vi "VisionUI.vi"() -> ()   [LabVIEW 2019]
uses:
  Ctrl/Snap.ctl
  Ctrl/Grab.ctl
  Ctrl/VisionProcessName.ctl
  Ctrl/UpDate.ctl
  Ctrl/Photo.ctl
  iVision/Analysis/Controls/V_Analysis_Type.ctl
  Ctrl/Calibration2.ctl
  <vilib>/vision/Image Controls.llb/IMAQ Image.ctl
  <vilib>/Utility/miscctls.llb/LVPointTypeDef.ctl
  <vilib>/Utility/miscctls.llb/LVPositionTypeDef.ctl
  iVision/Controls/Parameter.ctl
  LLB/Message/Ctrl/MsgDataInput.ctl
  LLB/Message/Ctrl/MsgPageSelect.ctl
  LLB/Message/Ctrl/LogType.ctl
  ccd1199d-ef2c-458d-9c2f-56e76543a288.vi
  ee1b8d73-df58-408e-9e82-1fda4488e2bc.vi
  7c6cd57d-ca9a-43cf-ba35-76cd5e228dea.vi
  c26e9516-a3f7-4664-a029-1caed30bc8c5.vi
  1dbde9c2-a06a-4c94-bdcc-a34a29a424c7.vi
  0675717f-6bf9-442b-96fb-61433deac2ff.vi
  bb48f479-1741-454e-9e2e-b2767c3551b8.vi
  488a8706-5b30-4d61-98bf-6c761bf059b6.vi
  687379a0-31af-4f7e-a561-925614dc81ac.vi
  a72d5238-090f-4a71-aba8-2c37060f7c47.vi
  74253ac0-82c8-4d34-a7ac-78c8919cb84d.vi
  340a900b-8271-4ea1-897c-4e5630e46489.vi
  8373cba2-dfce-4ae2-bf55-a53a2c69f5d3.vi
  <vilib>/JDP Science/JSONtext/Variant to JSON Text.vi
  LLB/Commonly VI/Main Glb.vi
  iVision/Global/VisionGlb.vi
  Class/Main Process Class/MPC_VirbVision/Panel RefGlb.vi
  <vilib>/JDP Science/JSONtext/JSON text to Variant.vi
  LLB/Commonly VI.lvlib
  <vilib>/vision/NI_Vision_Development_Module.lvlib
  LLB/Message/MsgShowAndLog.lvlib
panel:
  in  "Btn_Result Remove":bool
  in  "Btn_ResultAdd":bool
  in  "OutPutList":i32(listbox) caption="輸出列表"
  in  "Btn_Calibration":T1
  out "Calibration Axis Info":T2={"Origin Pixel"={"X"=0.0, "Y"=0.0}, "Angle Relative to Horizontal (deg)"=0.0, "X Axis Pixel"={"X"=0.0, "Y"=0.0}, "Axis Reference"=1} {"X Axis Pixel"."Y" format="%.2f"; "X Axis Pixel"."X" format="%.2f"; "Axis Reference" items=["Direct", "Indirect"]; "Angle Relative to Horizontal (deg)" format="%.2f"; "Origin Pixel"."Y" format="%.2f"; "Origin Pixel"."X" format="%.2f"}
  out "Grid Descriptor":T3={"X Step"=1.0, "Y Step"=1.0, "Unit"=enum."Undefined"} {"Y Step" format="%.2f"; "X Step" format="%.2f"}
  out "Calibration Done":bool
  in  "Btn_RemoveAlgorithm":bool
  in  "Btn_Add Algorithm":bool
  in  "AlgParameter":string
  in  "Algorithm List":i32(listbox)
  in  "SubUI":bool=TRUE
  out "PreProcess2":T5=enum."G_Threshold"
  in  "Btn_Load":bool
  out "Root Path":path
  in  "DataTable":T6(array[cluster])
  in  "Enum_Algorithm":enum16{"CG_Histogram", "C_Color Matching"}(ring)
  in  "Tab Control":enum32{"Page 1", "Page 2"}(tab)
  in  "Btn_ROITryrun":bool
  in  "Tab Control 3":enum32{"SetProcess", "ROI結果"}(tab)
  in  "Tab Control 2":enum32{"Process", "Algorithm", "Result"}(tab)
  in  "Btn_Test":bool
  out "Image 2":T7(plugin-control)
  in  "Enum_PreProcess":T5
  in  "Btn_RemovePreProcess":bool
  in  "Btn_Add PreProcess":bool
  in  "Process List":i32(listbox)
  in  "Algorithm":T8=enum."C_Color Pattern Matching"
  out "Image 3":T7(plugin-control)
  in  "Btn_TestAlg":bool
  in  "Btn_SetAlg":bool
  in  "Result":i32(listbox) caption="結果清單"
  in  "Btn_RenewROIData":T9
  in  "ROIOutPutList All":i32(listbox) caption="全部結果"
  in  "Photo":T10
  in  "Btn_DelProject":bool
  in  "Btn_AddProject":bool
  in  "Btn_EditROI":bool
  in  "Btn_DelROI":bool
  in  "Btn_AddROI":bool
  in  "btn_Grab":T11
  in  "Btn_Snap":T12
  in  "List ROI":i32(listbox)
  in  "Btn_Save":bool
  in  "ProjectSet":u16(ring) caption="設定資料"
  out "Image":T7(plugin-control)
  in  "相機":u16(ring) items=["cam0"]
  # "P_:Pixel\nR_RealWord"
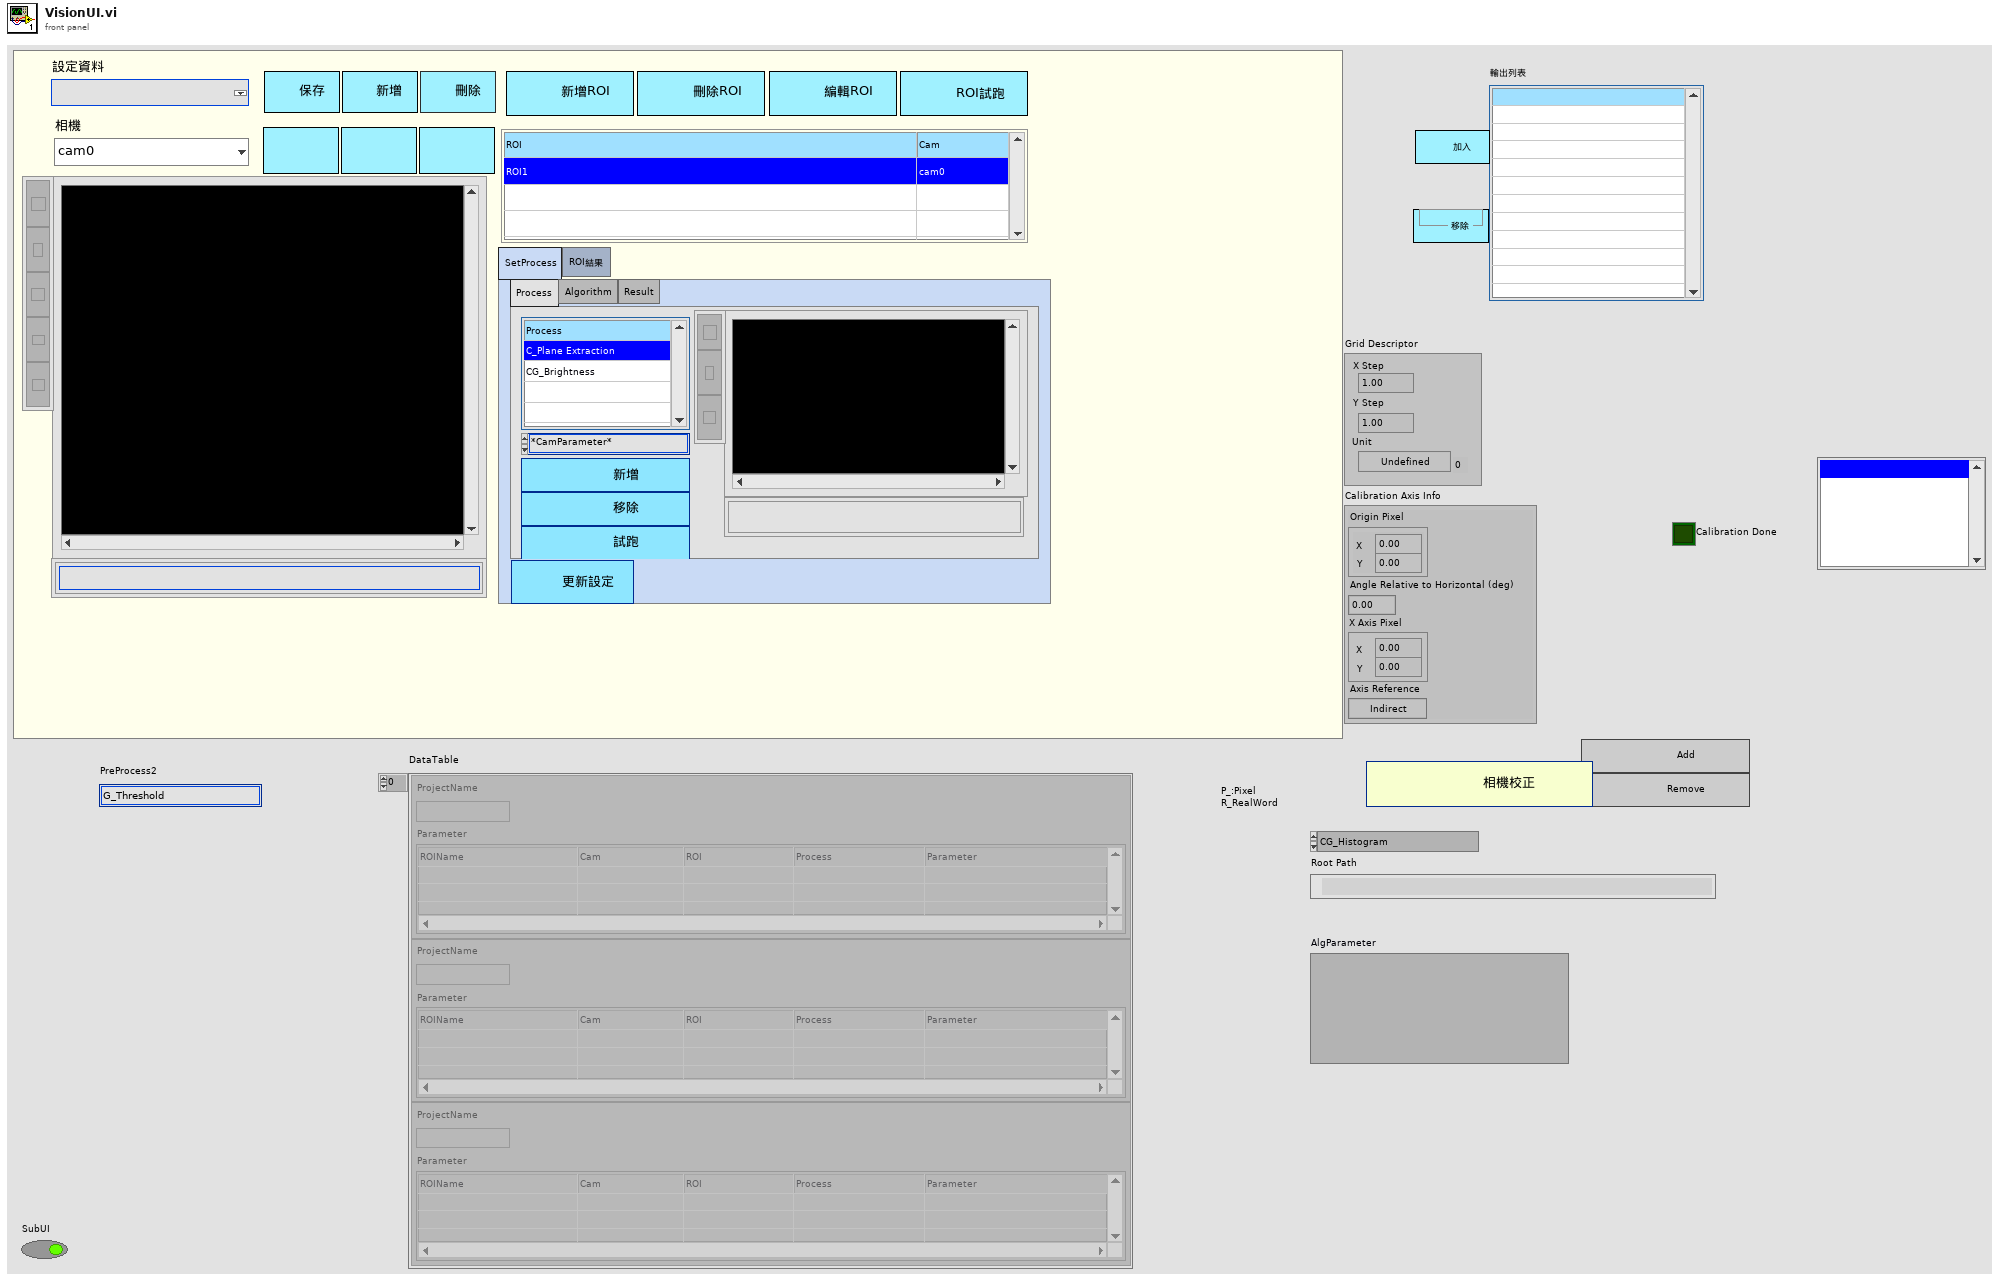
[diagram p1: front panel]
types:
  T1 = typedef "Calibration2.ctl" = bool
  T2 = cluster{"Origin Pixel":cluster{"X":sgl, "Y":sgl}, "Angle Relative to Horizontal (deg)":sgl, "X Axis Pixel":cluster{"X":sgl, "Y":sgl}, "Axis Reference":u32}
  T3 = typedef "Simple Grid Descriptor" = cluster{"X Step":sgl, "Y Step":sgl, "Unit":T4}
  T4 = typedef "Image Unit" = enum32{"Undefined", "Angström", "Micrometer", "Millimeter", "Centimeter", "Meter", "Kilometer", "Microinch", "Inch", "Feet", "Nautical miles", "Standard miles", "Steps"}
  T5 = typedef "VisionProcessName.ctl" = enum16{"*CamParameter*", "CamAttributes", "*Preprocess*", "CG_Brightness", "C_Plane Extraction", "C_Threshold", "G_Lookup Table", "G_Threshold"}
  T6 = cluster{"ProjectName":string, "Parameter":string[][]}[]
  T7 = typedef "IMAQ Image.ctl" = refnum<image>
  T8 = typedef "V_Analysis_Type.ctl" = enum16{"None", "C_Color Pattern Matching", "G_PatternMatching", "G_ShapeDectect", "G_GeometricMatch", "B_Area Check"}
  T9 = typedef "UpDate.ctl" = bool
  T10 = typedef "Photo.ctl" = bool
  T11 = typedef "Grab.ctl" = bool
  T12 = typedef "Snap.ctl" = bool
  T13 = typedef "MsgDataInput.ctl" = cluster{"MsgPageSelect":T14, "LogType":T15, "Msg":string, "Time":string}
  T14 = typedef "MsgShowAndLog.lvlib/MsgPageSelect.ctl" = enum16{"System", "Comm", "IO", "Action", "Alarm"}
  T15 = typedef "MsgShowAndLog.lvlib/LogType.ctl" = enum16{"Auto", "Manual", "Handshake", "Error"}
  T16 = cluster{"ProjectName":string, "Parameter":string[][]}
  T17 = enum16{"initial", "write", "add", "delete", "Load", "Save", "Read", "ReadProjectName"}
  T18 = typedef "LVPositionTypeDef.ctl" = cluster{"Left":i32, "Top":i32}
  T19 = typedef "LVPointTypeDef.ctl" = cluster{"Horizontal":i16, "Vertical":i16}
  T20 = enum16{"Init", "Grab", "Get All", "Close", "Set Camera"}
  T21 = typedef "Parameter.ctl" = enum16{"Initialize", "Write", "Read", "WriteAll", "Save", "Load"}
  T22 = enum8{"Enabled", "Disabled", "Disabled and Grayed Out"}
  T23 = cluster{"Real Points Valid?":bool, "Real Position":cluster{"X":dbl, "Y":dbl}[]}
  T24 = typedef "Image Type" = u32
  T25 = cluster{"Global Rectangle":i32[], "Contours":cluster{"Contour Type":u32, "ROI Type":u32, "Points":i32[]}[]}
  T26 = enum32{"invalid app kind", "Development System", "Run Time System", "Student Edition", "Embedded LabVIEW", "Evaluation", "Custom"}
  T27 = typedef "ParameterData.ctl" = cluster{"Rotate Angle":dbl, "Rotate?":bool, "Calibration File Path":string, "Cal?":bool}
  T28 = cluster{"RingText.Text":string, "ItemNames":string[][]}
  T29 = typedef "ROI Descriptor" = cluster{"Global Rectangle":i32[], "Contours":cluster{"ID":enum32{"External", "Internal"}, "Type":u32, "Coordinates":i32[]}[]}
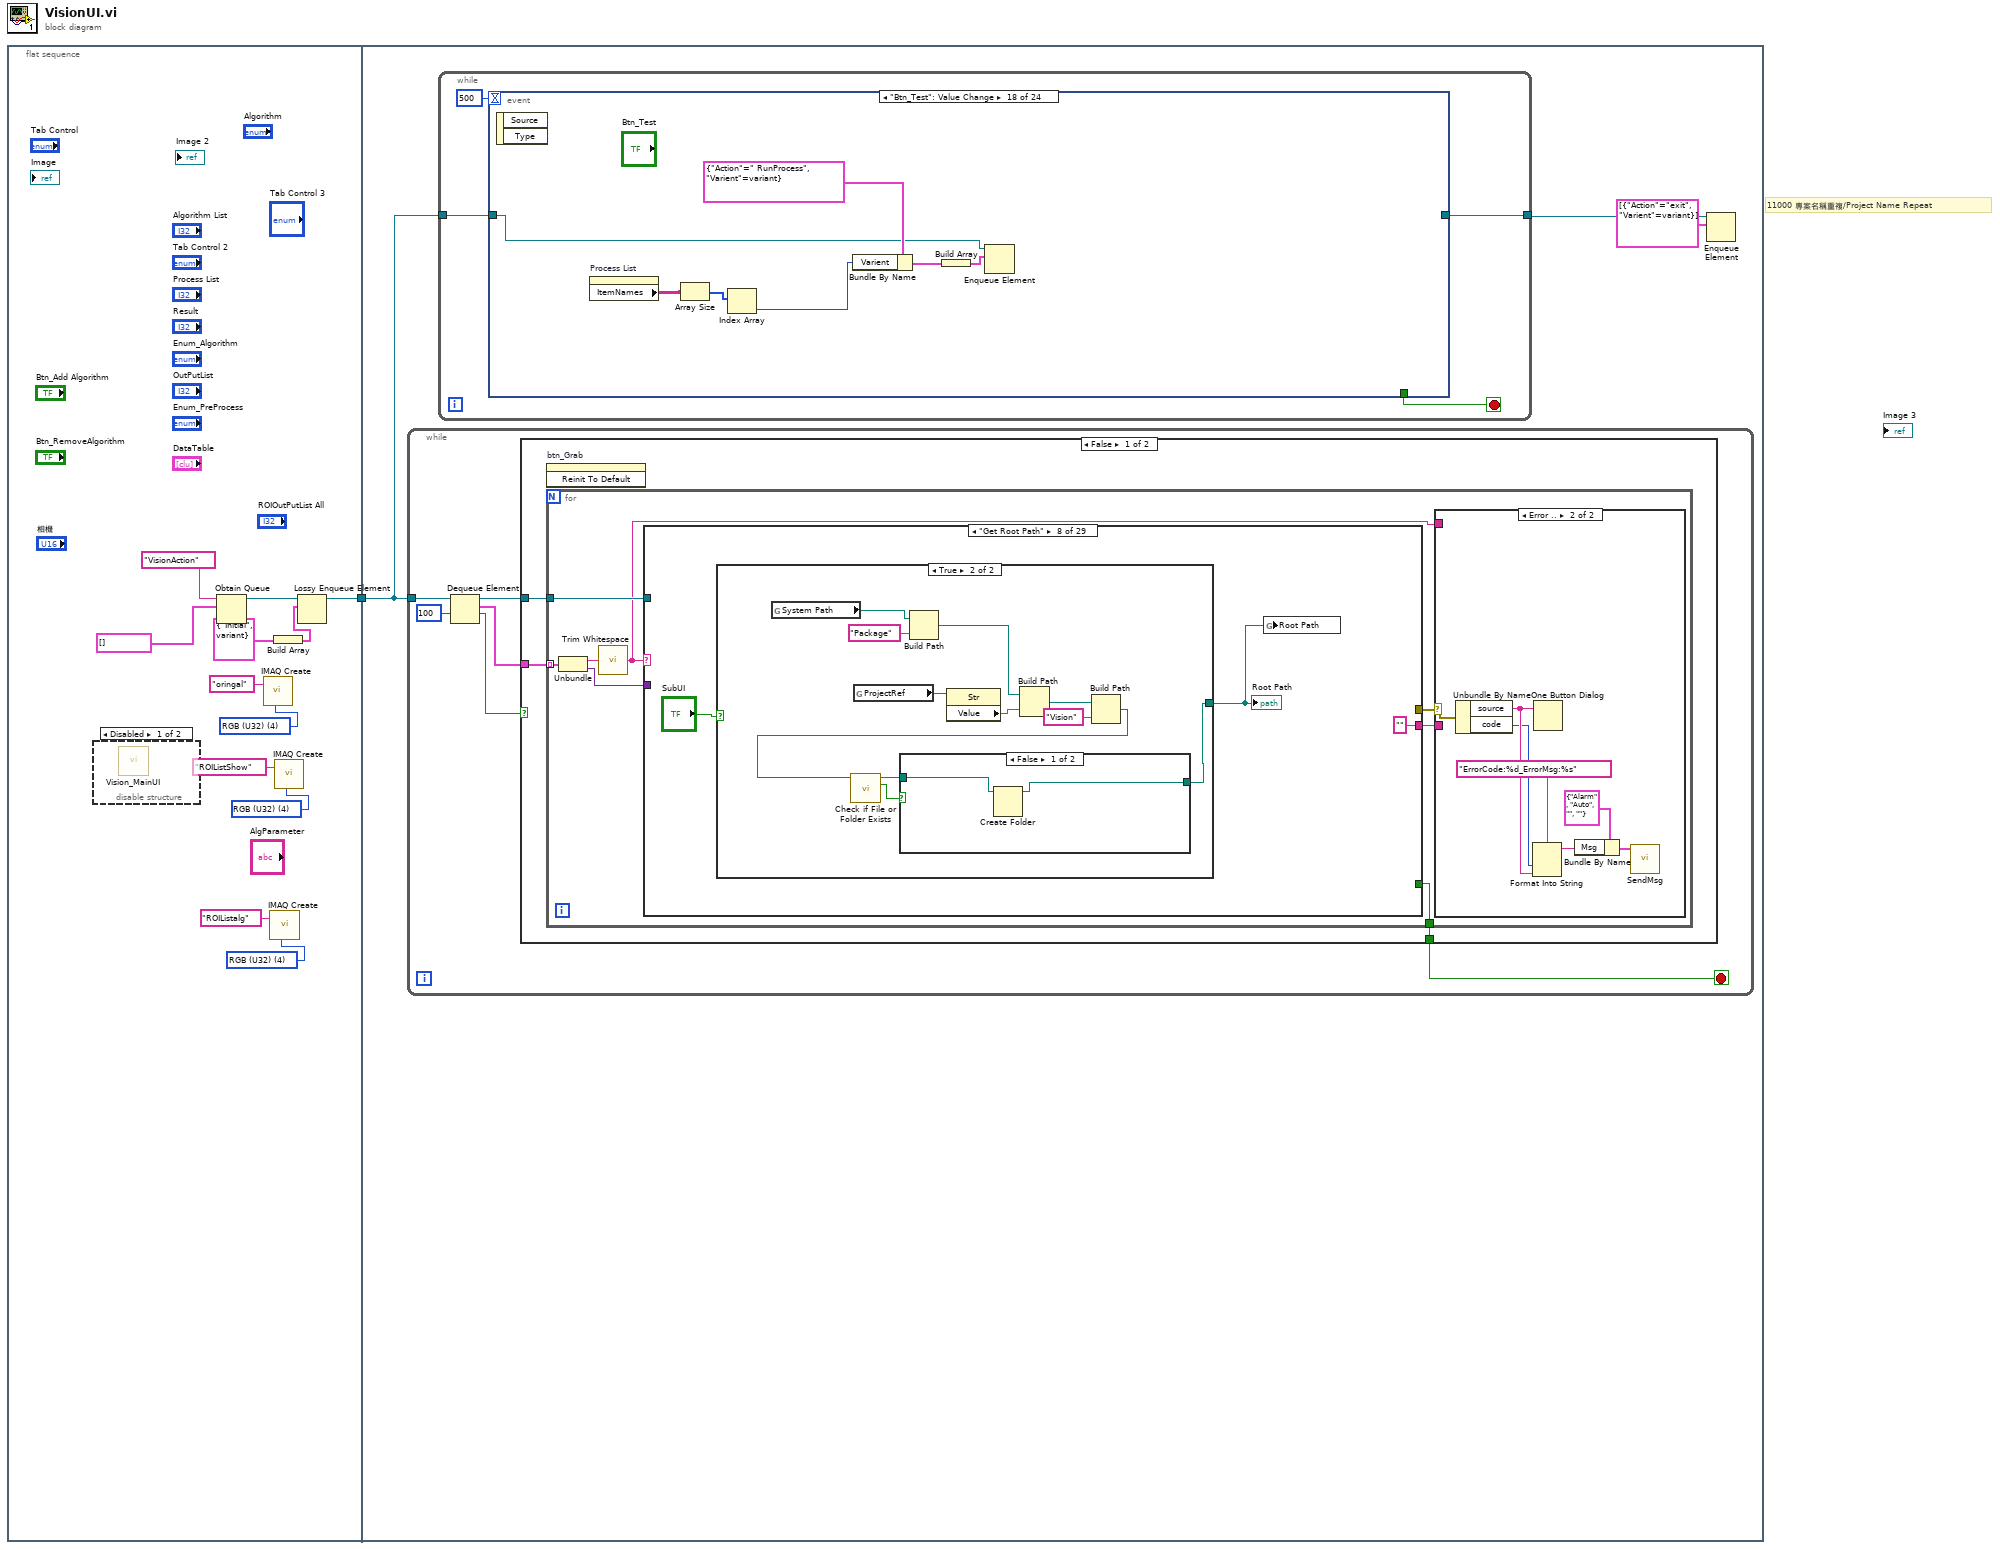
[diagram p0: block diagram]
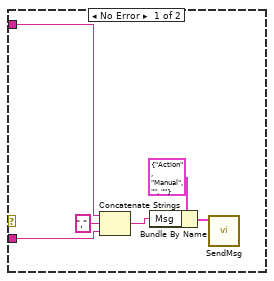
[diagram p3: hidden frame]
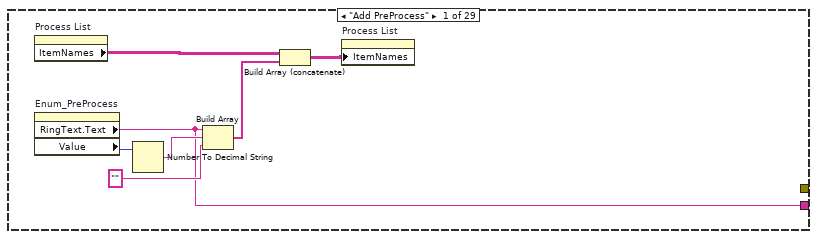
[diagram p4: hidden frame]
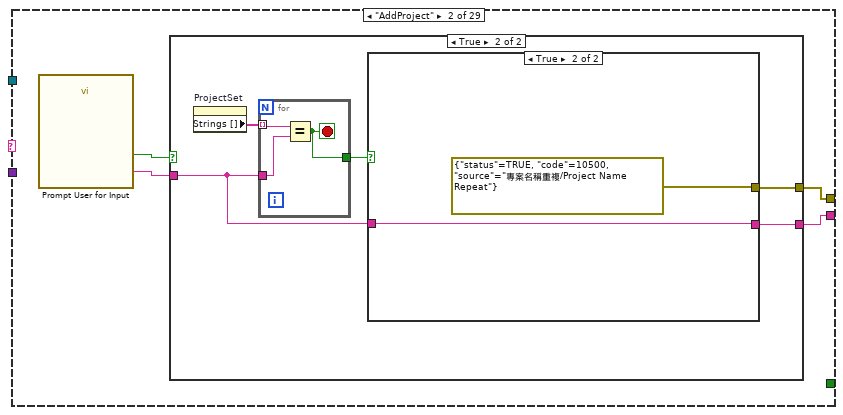
[diagram p5: hidden frame]
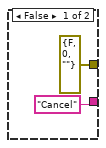
[diagram p6: hidden frame]
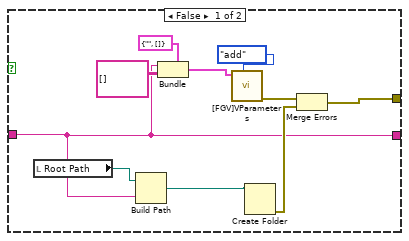
[diagram p7: hidden frame]
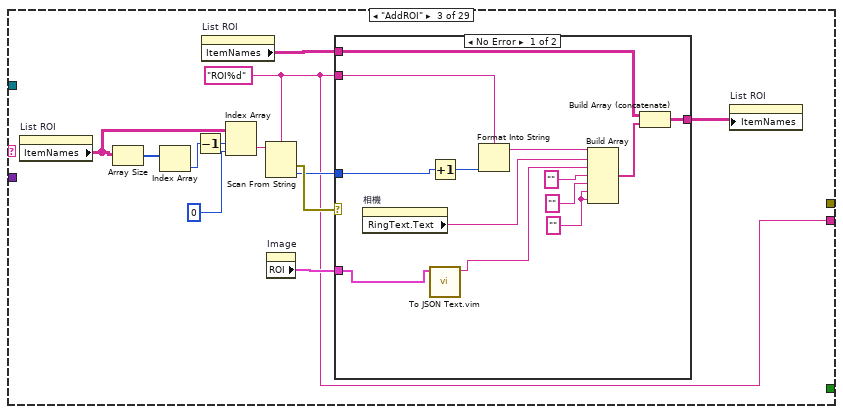
[diagram p8: hidden frame]
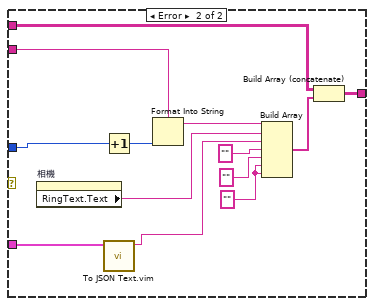
[diagram p9: hidden frame]
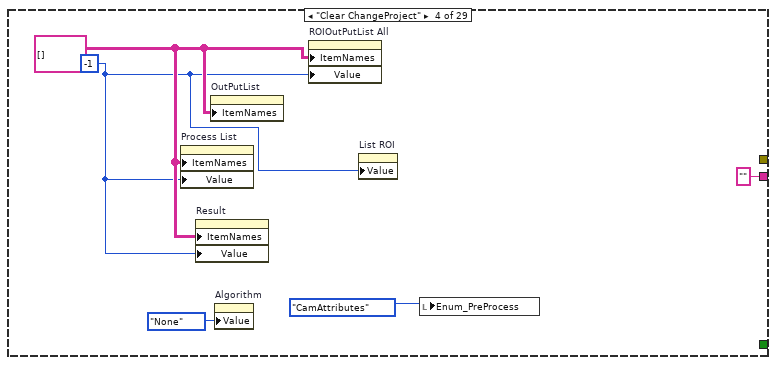
[diagram p10: hidden frame]
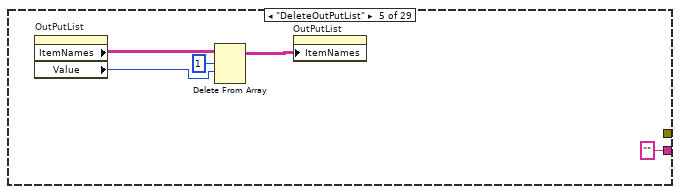
[diagram p11: hidden frame]
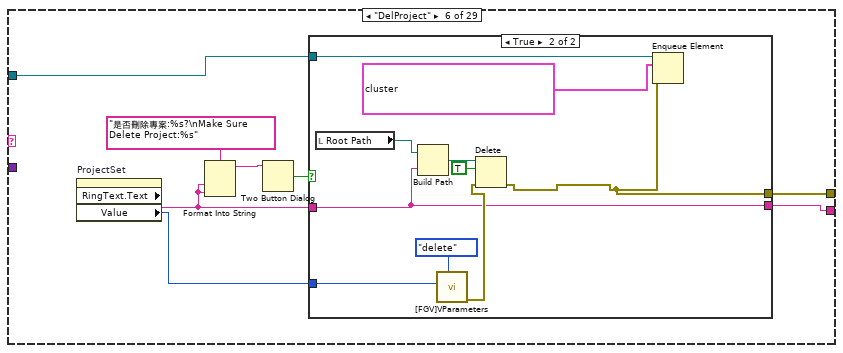
[diagram p12: hidden frame]
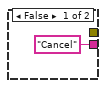
[diagram p13: hidden frame]
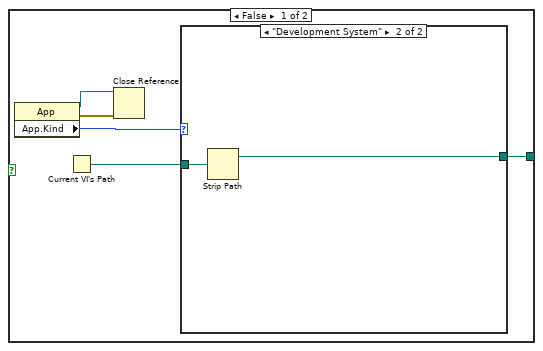
[diagram p15: hidden frame]
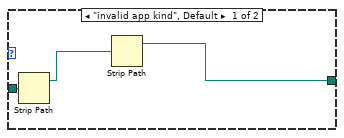
[diagram p16: hidden frame]
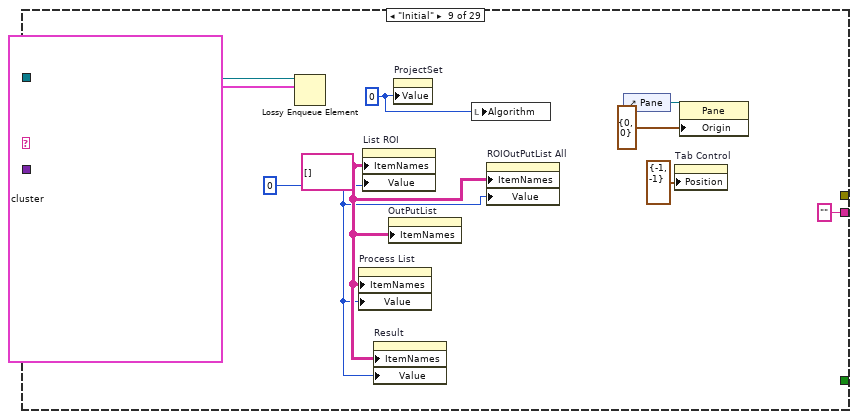
[diagram p18: hidden frame]
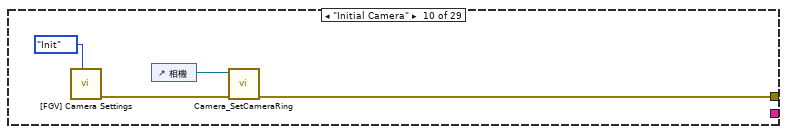
[diagram p19: hidden frame]
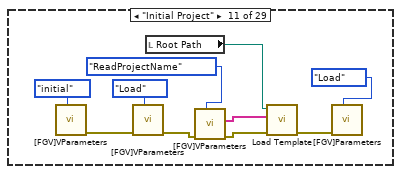
[diagram p20: hidden frame]
diagram:
  # "11000 專案名稱重複/Project Name Repeat"
  n1 = flat-sequence {
    tunnel: [w11] -> w1
    tunnel: w1 -> [w16]
    frame #0 {
      w2 = T24 4 items=["Grayscale (U8)", "Grayscale (I16)", "Grayscale (SGL)", "Complex (CSG)", "RGB (U32)", "HSL (U32)", "RGB (U64)", "Grayscale (U16)"] ("Image Type")
      w5 = T24 4 items=["Grayscale (U8)", "Grayscale (I16)", "Grayscale (SGL)", "Complex (CSG)", "RGB (U32)", "HSL (U32)", "RGB (U64)", "Grayscale (U16)"] ("Image Type")
      w6 = T24 4 items=["Grayscale (U8)", "Grayscale (I16)", "Grayscale (SGL)", "Complex (CSG)", "RGB (U32)", "HSL (U32)", "RGB (U64)", "Grayscale (U16)"] ("Image Type")
      n2 = disable-structure shown="Disabled" {
        frame Disabled {
          n3 = call "Vision_MainUI.vi"() -> ()  [unwired: 11 in, 1 out]
        }
        frame Enabled {
        }
      }
      n4 = Obtain Queue(name (unnamed)="VisionAction", element data type=cluster{"Action":string, "Varient":variant}[] []) -> (queue out=w12:refnum<queue>)  [unwired: 3 in, 2 out]
      n5 = call "IMAQ Create"("Image Name"="oringal", "Image Type"=w6) -> ()  [unwired: 3 in, 2 out]
      n6 = call "IMAQ Create"("Image Name"="ROIListalg", "Image Type"=w2) -> ()  [unwired: 3 in, 2 out]
      n7 = Build Array(cluster{"Action":string, "Varient":variant} {"Action"="Initial", "Varient"=variant} ("element")) -> (w8:cluster{"Action":string, "Varient":variant}[])
      n8 = call "IMAQ Create"("Image Name"="ROIListShow", "Image Type"=w5) -> ()  [unwired: 3 in, 2 out]
      n9 = Lossy Enqueue Element(queue=w12, element=w8) -> (queue out=w11:refnum<queue>)  [unwired: 1 in, 3 out]
    }
    frame #1 {
      n10 = while {
        tunnel: w16 -> [w22]
        stop <- w19 stop-if-true
        n11 = Dequeue Element(queue=w22, timeout in ms (-1)=100) -> (queue out=w20:refnum<queue>, element=w21:cluster{"Action":string, "Varient":variant}[], timed out?=w18:bool)  [unwired: 1 in, 1 out]
        n12 = case shown="False" w18 {
          tunnel: w21 -> [w25 _]
          tunnel: w20 -> [w24 _]
          tunnel: [w23 FALSE ("ExitOut")] -> w19
          frame False {
            n13 = invoke on="btn_Grab" class="Bool (strict)" method="Reinit To Default"() -> ()  [unwired: 3 in, 3 out]
            n14 = for {
              tunnel: w25 -> [w33] mode=indexing
              tunnel: w24 -> [w31]
              tunnel: [w29] -> w23
              n15 = Unbundle(w33) -> ("Action"=w32:string, "Varient"=w28:variant)
              n16 = call <vilib>:"Trim Whitespace.vi"("string"=w32) -> ("trimmed string"=w27:string)  [unwired: 1 in]
              n17 = case shown="\"Get Root Path\"" w27 {
                tunnel: w31 -> [_ _ _ _ _ w128 _ _ w182 _ _ _ _ _ _ _ _ _ _ _ _ _ _ _ _ _ _ _ _]
                tunnel: [_ w55 _ _ _ w130 _ _ _ w186 _ _ _ w209 _ _ _ w278 w285 w293 _ _ _ w409 _ w434 _ _ _] -> w30
                tunnel: [_ _ _ _ _ _ _ _ _ _ _ _ _ _ _ _ _ _ _ _ _ _ _ _ _ _ _ _ w459] -> w29
                tunnel: w28 -> [_ _ _ _ _ _ _ _ _ _ _ _ _ _ _ _ _ _ w291 _ _ _ _ _ _ _ _ _ _]
                tunnel: [w47 w54 w80 "" ("format string") "" ("format string") w129 _ "" ("RingText.Text") "" ("RingText.Text") _ _ _ _ w208 w225 w232 "" ("RingText.Text") w272 "" ("RingText.Text") "" ("RingText.Text") "" ("RingText.Text") w313 w371 w398 "" ("RingText.Text") "" ("RingText.Text") _ _ _] -> w26
                frame "Add PreProcess" {
                  n18 = property on="Process List" class="MCListbox (strict)"() -> ("ItemNames"=w53:string[][])  [unwired: 2 in, 2 out]
                  n19 = property on="Enum_PreProcess" class="Enum (strict)"() -> ("RingText.Text"=w47:string, "Value"=w51:T5)  [unwired: 2 in, 2 out]
                  n20 = Number To Decimal String(number=w51) -> (decimal integer string=w50:string)  [unwired: 1 in]
                  n21 = Build Array(w47, w50, "") -> (w48:string[])
                  n22 = Build Array (concatenate)(w53, w48) -> (w52:string[][])
                  n23 = property on="Process List" class="MCListbox (strict)"("ItemNames"=w52) -> ()  [unwired: 2 in, 2 out]
                }
                frame "AddProject" {
                  n24 = call "Prompt User for Input"() -> ("名稱/Name"=w57:string, "OK"=w56:bool)  [unwired: 17 in, 1 out]
                  n25 = case shown="True" w56 {
                    tunnel: w57 -> [_ w61]
                    tunnel: [errorcluster {"status"=FALSE, "code"=0, "source"=""} ("error constant") w62] -> w55
                    tunnel: ["Cancel" ("名稱/Name") w60] -> w54
                    frame False {
                    }
                    frame True {
                      n26 = property on="ProjectSet" class="Ring (strict)"() -> ("Strings []"=w64:string[])  [unwired: 2 in, 2 out]
                      n27 = for {
                        tunnel: w64 -> [w79] mode=indexing
                        tunnel: w61 -> [w78]
                        tunnel: [w77] -> w63
                        stop <- w77 stop-if-true
                        n28 = Equal?(x=w79, y=w78) -> (x = y?=w77:bool)
                      }
                      n29 = case shown="True" w63 {
                        tunnel: [w67 errorcluster {"status"=TRUE, "code"=10500, "source"="專案名稱重複/Project Name Repeat"} ("error constant")] -> w62
                        tunnel: w61 -> [w65 w75]
                        tunnel: [w65 w75] -> w60
                        frame False {
                          n30 = local read "Root Path"() -> (w68:path)
                          n31 = Build Path(base path=w68, name or relative path=w65) -> (appended path=w69:path)
                          n32 = Bundle(cluster=T16 {"ProjectName"="", "Parameter"=[]} ("DataIn"), "ProjectName"=w65, "Parameter"=string[][] []) -> (w71:T16)
                          n33 = call "[FGV]VParameters.vi"("Enum"=T17."add", "DataIn"=w71) -> ("error out"=w73:errorcluster)  [unwired: 6 in, 3 out]
                          n34 = Create Folder(path (use dialog)=w69) -> (error out=w66:errorcluster)  [unwired: 2 in, 2 out]
                          n35 = Merge Errors(w73, w66) -> (w67:errorcluster)
                        }
                        frame True {
                        }
                      }
                    }
                  }
                }
                frame "AddROI" {
                  w80 = "ROI%d" ("format string")
                  n36 = property on="List ROI" class="MCListbox (strict)"() -> ("ItemNames"=w90:string[][])  [unwired: 2 in, 2 out]
                  n37 = Array Size(array=w90) -> (size(s)=w91:i32[])
                  n38 = Index Array(array=w91) -> (element=w88:i32)  [unwired: 1 in]
                  n39 = Decrement(x=w88) -> (x-1=w81:i32)
                  n40 = property on="List ROI" class="MCListbox (strict)"() -> ("ItemNames"=w83:string[][])  [unwired: 2 in, 2 out]
                  n41 = Index Array(array=w90, index (row)=w81, index (col)=0 ("disabled index (col)")) -> (element=w87:string)
                  n42 = Scan From String(format string=w80, input string=w87) -> (error out=w86:errorcluster, output 1=w85:i32)  [unwired: 3 in, 2 out]
                  n43 = property on="Image" class="ImageControl"() -> ("ROI"=w84:T25)  [unwired: 2 in, 2 out]
                  n44 = case shown="No Error" w86 {
                    tunnel: w80 -> [w97 w110]
                    tunnel: w85 -> [w96 w106]
                    tunnel: w84 -> [w93 w109]
                    tunnel: w83 -> [w95 w108]
                    tunnel: [w94 w107] -> w82
                    frame No Error {
                      w92 = ""
                      n45 = property on="相機" class="Ring (strict)"() -> ("RingText.Text"=w102:string)  [unwired: 2 in, 2 out]
                      n46 = Increment(x=w96) -> (x+1=w104:i32)
                      n47 = call "To JSON Text.vim"("Anything"=w93) -> ("<JSON>"=w101:string)  [unwired: 9 in, 1 out]
                      n48 = Format Into String(format string=w97, w104) -> (resulting string=w103:string)  [unwired: 2 in, 1 out]
                      n49 = Build Array(w103, w102, w101, "", "", w92, w92) -> (w98:string[])
                      n50 = Build Array (concatenate)(w95, w98) -> (w94:string[][])
                    }
                    frame Error {
                      w105 = ""
                      n51 = property on="相機" class="Ring (strict)"() -> ("RingText.Text"=w115:string)  [unwired: 2 in, 2 out]
                      n52 = Increment(x=w106) -> (x+1=w117:i32)
                      n53 = call "To JSON Text.vim"("Anything"=w109) -> ("<JSON>"=w114:string)  [unwired: 9 in, 1 out]
                      n54 = Format Into String(format string=w110, w117) -> (resulting string=w116:string)  [unwired: 2 in, 1 out]
                      n55 = Build Array(w116, w115, w114, "", "", w105, w105) -> (w111:string[])
                      n56 = Build Array (concatenate)(w108, w111) -> (w107:string[][])
                    }
                  }
                  n57 = property on="List ROI" class="MCListbox (strict)"("ItemNames"=w82) -> ()  [unwired: 2 in, 2 out]
                }
                frame "Clear ChangeProject" {
                  w120 = -1 ("List ROI")
                  w122 = string[][] [] ("Item Names")
                  n58 = property on="Process List" class="MCListbox (strict)"("ItemNames"=w122, "Value"=w120) -> ()  [unwired: 2 in, 2 out]
                  n59 = property on="Result" class="MCListbox (strict)"("ItemNames"=w122, "Value"=w120) -> ()  [unwired: 2 in, 2 out]
                  n60 = property on="OutPutList" class="MCListbox (strict)"("ItemNames"=w122) -> ()  [unwired: 2 in, 2 out]
                  n61 = property on="Algorithm" class="Enum (strict)"("Value"=V_Analysis_Type."None" ("Algorithm")) -> ()  [unwired: 2 in, 2 out]
                  n62 = property on="ROIOutPutList All" class="MCListbox (strict)"("ItemNames"=w122, "Value"=w120) -> ()  [unwired: 2 in, 2 out]
                  n63 = property on="List ROI" class="MCListbox (strict)"("Value"=w120) -> ()  [unwired: 2 in, 2 out]
                  n64 = local write "Enum_PreProcess"(VisionProcessName."CamAttributes" ("Enum_PreProcess")) -> ()
                }
                frame "DeleteOutPutList" {
                  n65 = property on="OutPutList" class="MCListbox (strict)"() -> ("ItemNames"=w127:string[][], "Value"=w125:i32)  [unwired: 2 in, 2 out]
                  n66 = Delete From Array(array=w127, length=1, index (row)=w125) -> (array with subset deleted=w124:string[][])  [unwired: 1 in, 1 out]
                  n67 = property on="OutPutList" class="MCListbox (strict)"("ItemNames"=w124) -> ()  [unwired: 2 in, 2 out]
                }
                frame "DelProject" {
                  n68 = property on="ProjectSet" class="Ring (strict)"() -> ("RingText.Text"=w132:string, "Value"=w131:u16)  [unwired: 2 in, 2 out]
                  n69 = Format Into String(format string="是否刪除專案:%s?\nMake Sure Delete Project:%s", w132, w132) -> (resulting string=w134:string)  [unwired: 2 in, 1 out]
                  n70 = Two Button Dialog(message=w134) -> (T button?=w133:bool)  [unwired: 2 in]
                  n71 = case shown="True" w133 {
                    tunnel: w132 -> [_ w140]
                    tunnel: w131 -> [_ w143]
                    tunnel: [_ w137] -> w130
                    tunnel: ["Cancel" ("RingText.Text") w140] -> w129
                    tunnel: w128 -> [_ w139]
                    frame False {
                    }
                    frame True {
                      n72 = local read "Root Path"() -> (w146:path)
                      n73 = Build Path(base path=w146, name or relative path=w140) -> (appended path=w145:path)
                      n74 = call "[FGV]VParameters.vi"("Enum"=T17."delete", "ProjectIndex"=w143) -> ("error out"=w142:errorcluster)  [unwired: 6 in, 3 out]
                      n75 = Delete(path (use dialog)=w145, entire hierarchy (F)=TRUE, error in=w142) -> (error out=w137:errorcluster)  [unwired: 2 in, 2 out]
                      n76 = Enqueue Element(queue=w139, element=cluster{"Action":string, "Varient":variant}[] [{"Action"="UpdateProjectSet", "Varient"=variant}, {"Action"="UpDateDataToList ROI", "Varient"=variant}, {"Action"="Clear ChangeProject ", "Varient"=variant}], error in (no error)=w137) -> ()  [unwired: 1 in, 3 out]
                    }
                  }
                }
                frame "False", Default {
                }
                frame "Get Root Path" {
                  n77 = case shown="True" "SubUI" {
                    tunnel: [w150 w161] -> w149
                    frame False {
                      n78 = property class="App"() -> (reference out=w151:refnum<vi>, error out=w152:errorcluster, "App.Kind"=w154:T26)  [unwired: 2 in]
                      n79 = Current VI's Path() -> (path=w153:path)
                      n80 = Close Reference(reference=w151, error in (no error)=w152) -> ()  [unwired: 1 out]
                      n81 = case shown="\"Development System\"" w154 {
                        tunnel: w153 -> [w157 w159]
                        tunnel: [w155 w158] -> w150
                        frame "invalid app kind", Default {
                          n82 = Strip Path(path=w157) -> (stripped path=w156:path)  [unwired: 1 out]
                          n83 = Strip Path(path=w156) -> (stripped path=w155:path)  [unwired: 1 out]
                        }
                        frame "Development System" {
                          n84 = Strip Path(path=w159) -> (stripped path=w158:path)  [unwired: 1 out]
                        }
                      }
                    }
                    frame True {
                      n85 = global read "Main Glb.vi" "System Path"() -> (w168:path)
                      n86 = global read "Main Glb.vi" "ProjectRef"() -> (w170:refnum<vi>)
                      n87 = Build Path(base path=w168, name or relative path="Package") -> (appended path=w167:path)
                      n88 = property class="Str"(reference=w170) -> ("Value"=w169:string)  [unwired: 1 in, 2 out]
                      n89 = Build Path(base path=w167, name or relative path=w169) -> (appended path=w165:path)
                      n90 = Build Path(base path=w165, name or relative path="Vision") -> (appended path=w163:path)
                      n91 = call <vilib>:"Check if File or Folder Exists.vi"("path"=w163) -> ("file or folder exists?"=w162:bool, "dup path"=w160:path)  [unwired: 8 in, 1 out]
                      n92 = case shown="False" w162 {
                        tunnel: [w171 w173] -> w161
                        tunnel: w160 -> [w172 w173]
                        frame False {
                          n93 = Create Folder(path (use dialog)=w172) -> (created path=w171:path)  [unwired: 2 in, 2 out]
                        }
                        frame True {
                        }
                      }
                    }
                  }
                  "Root Path" <- w149
                  n94 = global write "VisionGlb.vi" "Root Path"(w149) -> ()
                }
                frame "Initial" {
                  w178 = 0 ("List ROI")
                  w179 = string[][] [] ("Item Names")
                  w180 = 0
                  n95 = Lossy Enqueue Element(queue=w182, element=cluster{"Action":string, "Varient":variant}[] [{"Action"="Get Root Path", "Varient"=variant}, {"Action"="Initial Project", "Varient"=variant}, {"Action"="UpdateProjectSet", "Varient"=variant}, {"Action"="UpDateDataToList ROI", "Varient"=variant}, {"Action"="Initial Camera", "Varient"=variant}]) -> ()  [unwired: 1 in, 4 out]
                  n96 = property on="Process List" class="MCListbox (strict)"("ItemNames"=w179, "Value"=w178) -> ()  [unwired: 2 in, 2 out]
                  n97 = property on="List ROI" class="MCListbox (strict)"("ItemNames"=w179, "Value"=w178) -> ()  [unwired: 2 in, 2 out]
                  n98 = property on="Result" class="MCListbox (strict)"("ItemNames"=w179, "Value"=w178) -> ()  [unwired: 2 in, 2 out]
                  n99 = property on="OutPutList" class="MCListbox (strict)"("ItemNames"=w179) -> ()  [unwired: 2 in, 2 out]
                  n100 = property on="ProjectSet" class="Ring (strict)"("Value"=w180) -> ()  [unwired: 2 in, 2 out]
                  n101 = local write "Algorithm"(w180) -> ()
                  n102 = property on="ROIOutPutList All" class="MCListbox (strict)"("ItemNames"=w179, "Value"=w178) -> ()  [unwired: 2 in, 2 out]
                  n103 = control-ref of="Pane"() -> (w177:refnum<vi>)
                  n104 = property on="Tab Control" class="TabCtl (strict)"("Position"=T18 {"Left"=-1, "Top"=-1}) -> ()  [unwired: 2 in, 2 out]
                  n105 = property class="Pane"(reference=w177, "Origin"=T19 {"Horizontal"=0, "Vertical"=0}) -> ()  [unwired: 1 in, 2 out]
                }
                frame "Initial Camera" {
                  n106 = call "[FGV] Camera Settings.vi"("Action"=T20."Init") -> ("error out"=w183:errorcluster)  [unwired: 8 in, 2 out]
                  n107 = control-ref of="相機"() -> (w184:refnum<vi>)
                  n108 = call "Camera_SetCameraRing.vi"("error in (no error)"=w183, "CameraName"=w184) -> ("error out"=w186:errorcluster)  [unwired: 9 in]
                }
                frame "Initial Project" {
                  n109 = call "[FGV]VParameters.vi"("Enum"=T17."initial") -> ("error out"=w194:errorcluster)  [unwired: 7 in, 3 out]
                  n110 = call "[FGV]VParameters.vi"("Enum"=T17."Load", "error in"=w194) -> ("error out"=w189:errorcluster)  [unwired: 6 in, 3 out]
                  n111 = local read "Root Path"() -> (w193:path)
                  n112 = call "[FGV]VParameters.vi"("Enum"=T17."ReadProjectName", "error in"=w189) -> ("error out"=w190:errorcluster, "ProjectName"=w191:string[])  [unwired: 6 in, 2 out]
                  n113 = call "Load Template.vi"("error in (no error)"=w190, "VisionProjectName"=w191, "root"=w193) -> ("error out"=w187:errorcluster)  [unwired: 8 in]
                  n114 = call "[FGV]Parameters.vi"("Parameter"=Parameter."Load", "Error In"=w187) -> ()  [unwired: 8 in, 2 out]
                }
                frame "loadfinish" {
                  n115 = global write "Panel RefGlb.vi" "vision load"(TRUE ("vision load")) -> ()
                }
                frame "OverlayROI" {
                  n116 = property on="List ROI" class="MCListbox (strict)"() -> ("ItemNames"=w206:string[][], "Value"=w205:i32)  [unwired: 2 in, 2 out]
                  n117 = local read "Image"() -> (w207:T7)
                  n118 = Index Array(array=w206, index (row)=w205, index (col)=2 ("disabled index (col)")) -> (element=w203:string)
                  n119 = call "IMAQ Clear Overlay"("Image"=w207) -> ("error out"=w199:errorcluster, "Image Out"=w201:T7)  [unwired: 9 in]
                  n120 = property on="Image" class="ImageControl"() -> ("ROI"=w202:T25)  [unwired: 2 in, 2 out]
                  n121 = call "From JSON Text.vim"("Data Type and Default Value"=w202, "JSON"=w203) -> ("Data out"=w200:T25)  [unwired: 8 in, 1 out]
                  n122 = call "IMAQ Overlay ROI"("error in (no error)"=w199, "ROI Descriptor"=w200, "Image"=w201) -> ("Image Out"=w198:T7)  [unwired: 7 in, 1 out]
                  n123 = local write "Image"(w198) -> ()
                }
                frame "Photo" {
                  n124 = call "File Dialog"("prompt"="選擇圖片/Select Picture", "pattern (all files)"="*.bmp;*.png;*.jpg;*.jpeg" ("pattern label")) -> ("selected path"=w211:path, "error out"=w212:errorcluster)  [unwired: 10 in, 2 out]
                  n125 = case shown="Error .." w212 {
                    tunnel: w211 -> [w214 _]
                    tunnel: [w218 errorcluster {"status"=FALSE, "code"=0, "source"=""} ("error out")] -> w209
                    tunnel: [w215 "Not Path"] -> w208
                    frame No Error {
                      w222 = T24 4 items=["Grayscale (U8)", "Grayscale (I16)", "Grayscale (SGL)", "Complex (CSG)", "RGB (U32)", "HSL (U32)", "RGB (U64)", "Grayscale (U16)"] ("Image Type")
                      n126 = call "IMAQ Create"("Image Name"="photo", "Image Type"=w222) -> ("New Image"=w220:T7, "error out"=w219:errorcluster)  [unwired: 3 in]
                      n127 = call "IMAQ ReadFile 2"("File Path"=w214, "error in (no error)"=w219, "Image"=w220) -> ("error out"=w218:errorcluster, "Image Out"=w216:T7)  [unwired: 4 in, 3 out]
                      n128 = local write "Image"(w216) -> ()
                      n129 = call "IMAQ Copy"("Image Dst"="oringal" ("Image Name"), "Image Src"=w216) -> ()  [unwired: 4 in, 2 out]
                      n130 = Path To String(path=w214) -> (string=w215:string)
                    }
                    frame Error {
                    }
                  }
                }
                frame "RemovePreProcess" {
                  w226 = 0 ("disabled index (col)")
                  n131 = property on="Process List" class="MCListbox (strict)"() -> ("ItemNames"=w231:string[][], "Value"=w229:i32)  [unwired: 2 in, 2 out]
                  n132 = Delete From Array(array=w231, length=1, index (row)=w229) -> (deleted portion=w227:string[][], array with subset deleted=w230:string[][])  [unwired: 1 in]
                  n133 = Index Array(array=w227, index (row)=w226, index (col)=w226) -> (element=w225:string)
                  n134 = property on="Process List" class="MCListbox (strict)"("ItemNames"=w230) -> ()  [unwired: 2 in, 2 out]
                }
                frame "RenewROIData" {
                  n135 = local read "AlgParameter"() -> (w243:string)
                  n136 = property on="Algorithm" class="Enum (strict)"() -> ("RingText.Text"=w245:string, "Value"=w246:T8)  [unwired: 2 in, 2 out]
                  n137 = property on="Process List" class="MCListbox (strict)"() -> ("ItemNames"=w250:string[][])  [unwired: 2 in, 2 out]
                  n138 = property on="Result" class="MCListbox (strict)"() -> ("ItemNames"=w239:string[][])  [unwired: 2 in, 2 out]
                  n139 = Number To Decimal String(number=w246) -> (decimal integer string=w244:string)  [unwired: 1 in]
                  n140 = call "To JSON Text.vim"("Anything"=w250) -> ("<JSON>"=w249:string)  [unwired: 9 in, 1 out]
                  n141 = Build Array(w245, w244, w243) -> (w242:string[])
                  n142 = property on="List ROI" class="MCListbox (strict)"() -> ("ItemNames"=w252:string[][], "Value"=w233:i32)  [unwired: 2 in, 2 out]
                  n143 = call "To JSON Text.vim"("Anything"=w239) -> ("<JSON>"=w238:string)  [unwired: 9 in, 1 out]
                  n144 = call "To JSON Text.vim"("Anything"=w242) -> ("<JSON>"=w247:string)  [unwired: 9 in, 1 out]
                  n145 = property on="OutPutList" class="MCListbox (strict)"() -> ("ItemNames"=w236:string[][])  [unwired: 2 in, 2 out]
                  n146 = call "To JSON Text.vim"("Anything"=w236) -> ("<JSON>"=w237:string)  [unwired: 9 in, 1 out]
                  n147 = Replace Array Subset(array=w252, new element #1=w249, index (row) #1=w233, index (col) #1=3 ("disabled index (col)"), new element #2=w247, index (row) #2=w233, index (col) #2=4 ("disabled index (col)"), new element #3=w238, index (row) #3=w233, index (col) #3=5 ("disabled index (col)"), new element #4=w237, index (row) #4=w233, index (col) #4=6 ("disabled index (col)")) -> (w235:string[][])
                  n148 = property on="List ROI" class="MCListbox (strict)"("ItemNames"=w235) -> ()  [unwired: 2 in, 2 out]
                  n149 = Index Array(array=w235, index (row)=w233, index (col)=0 ("disabled index (col)")) -> (element=w232:string)
                }
                frame "ResultAdd" {
                  n150 = property on="Result" class="MCListbox (strict)"() -> ("ItemNames"=w263:string[][], "Value"=w255:i32)  [unwired: 2 in, 2 out]
                  n151 = property on="OutPutList" class="MCListbox (strict)"() -> ("ItemNames"=w257:string[][])  [unwired: 2 in, 2 out]
                  n152 = Index Array(array=w263, index (row) #1=w255, index (col) #1=0 ("disabled index (col)"), index (row) #2=w255) -> (element #1=w256:string)  [unwired: 1 in, 1 out]
                  n153 = Index Array(array=w257, index (col)=0 ("disabled index (col)")) -> (element=w260:string[])  [unwired: 1 in]
                  n154 = Search 1D Array(1D array=w260, element=w256) -> (index of element=w259:i32)  [unwired: 1 in]
                  n155 = Number To Decimal String(number=w255) -> (decimal integer string=w254:string)  [unwired: 1 in]
                  n156 = Less Than 0?(x=w259) -> (x < 0?=w258:bool)
                  n157 = case shown="False" w258 {
                    tunnel: w257 -> [_ w269]
                    tunnel: w256 -> [_ w267]
                    tunnel: w254 -> [_ w265]
                    frame False {
                      n158 = One Button Dialog(message="該參數以加入輸出列表\nSelect Parameter Already Exist") -> ()  [unwired: 1 in, 1 out]
                    }
                    frame True {
                      n159 = Build Array(w267, w265) -> (w268:string[])
                      n160 = Build Array (concatenate)(w269, w268) -> (w266:string[][])
                      n161 = property on="OutPutList" class="MCListbox (strict)"("ItemNames"=w266) -> ()  [unwired: 2 in, 2 out]
                    }
                  }
                }
                frame "RunAlg" {
                  n162 = local read "AlgParameter"() -> (w277:string)
                  n163 = property on="List ROI" class="MCListbox (strict)"() -> ("ItemNames"=w280:string[][], "Value"=w279:i32)  [unwired: 2 in, 2 out]
                  n164 = local read "Image 2"() -> (w271:T7)
                  n165 = local read "Algorithm"() -> (w274:T8)
                  n166 = call "Total Analysis V.vi"("ROIIndex"=w279, "Algorithm"=w274, "ROIList"=w280, "AlgParameter"=w277, "Img in"=w271) -> ("error out"=w278:errorcluster, "DetectResult"=w273:variant, "ResultOut"=w276:string[][], "Img out"=w270:T7)  [unwired: 3 in]
                  n167 = call "OverlayResult.vi"("DectectResult"=w273, "Algorithm"=w274, "Image"=w270) -> ("Image Out"=w275:T7)  [unwired: 8 in]
                  n168 = property on="Result" class="MCListbox (strict)"("ItemNames"=w276) -> ()  [unwired: 2 in, 2 out]
                  n169 = local write "Image 3"(w275) -> ()
                  n170 = property on="Algorithm" class="Enum (strict)"() -> ("RingText.Text"=w272:string)  [unwired: 2 in, 2 out]
                }
                frame "RunProcess" {
                  n171 = property on="Process List" class="MCListbox (strict)"() -> ("ItemNames"=w289:string[][])  [unwired: 2 in, 2 out]
                  n172 = Variant To Data(type=0, Variant=w291) -> (data=w283:i32)  [unwired: 1 in, 1 out]
                  n173 = Array Size(array=w289) -> (size(s)=w288:i32[])
                  n174 = Index Array(array=w288) -> ()  [unwired: 1 in, 1 out]
                  n175 = Array Subset(array=w289, index (row)=0 ("index"), length (row)=w283) -> (w286:string[][])  [unwired: 2 in]
                  n176 = call "SingleImgProcess.vi"("Process List"=w286, "Refnum in"="oringal" ("Image Name")) -> ("error out"=w285:errorcluster, "ImgOut"=w284:T7)  [unwired: 8 in]
                  n177 = local write "Image 2"(w284) -> ()
                }
                frame "RunROIList" {
                  w296 = "oringal" ("Image Name")
                  n178 = property on="List ROI" class="MCListbox (strict)"() -> ("ItemNames"=w292:string[][])  [unwired: 2 in, 2 out]
                  n179 = call "IMAQ Copy"("Image Dst"="ROIListalg" ("Image Name"), "Image Src"=w296) -> ("Image Dst Out"=w298:T7)  [unwired: 4 in, 1 out]
                  n180 = call "Run Process And Alg.vi"("ROIList"=w292, "Image"=w298) -> ("DetectOut"=w302:variant[], "ALLResultOut"=w295:string[][], "AlgOut"=w301:i32[], "error out"=w293:errorcluster)  [unwired: 5 in, 1 out]
                  n181 = call "IMAQ Copy"("Image Dst"="ROIListShow" ("Image Name"), "Image Src"=w296) -> ("Image Dst Out"=w303:T7)  [unwired: 4 in, 1 out]
                  n182 = for {
                    tunnel: w302 -> [w306] mode=indexing
                    shift-right: [w305] -> w300
                    shift-left: w303 -> [w307]
                    tunnel: w301 -> [w304] mode=indexing
                    tunnel: w292 -> [_] mode=indexing
                    n183 = call "OverlayResult.vi"("DectectResult"=w306, "Algorithm"=w304, "Image"=w307) -> ("Image Out"=w305:T7)  [unwired: 8 in]
                  }
                  n184 = property on="ROIOutPutList All" class="MCListbox (strict)"("ItemNames"=w295) -> ()  [unwired: 2 in, 2 out]
                  n185 = local write "Image"(w300) -> ()
                }
                frame "SaveDataTable" {
                  n186 = property on="ProjectSet" class="Ring (strict)"() -> ("Value"=w310:u16)  [unwired: 2 in, 2 out]
                  n187 = call "[FGV]VParameters.vi"("Enum"=T17."Save", "ProjectIndex"=w310) -> ("error out"=w308:errorcluster)  [unwired: 6 in, 3 out]
                  n188 = flat-sequence {
                    tunnel: w308 -> [_]
                    frame #0 {
                      n189 = One Button Dialog(message="資料保存成功\n Data Save OK") -> ()  [unwired: 1 in, 1 out]
                    }
                  }
                }
                frame "SetAlgPanel" {
                  n190 = property on="ProjectSet" class="Ring (strict)"() -> ("RingText.Text"=w328:string)  [unwired: 2 in, 2 out]
                  n191 = local read "Image 2"() -> (w316:T7)
                  n192 = property on="List ROI" class="MCListbox (strict)"() -> ("ItemNames"=w322:string[][], "Value"=w321:i32)  [unwired: 2 in, 2 out]
                  n193 = local read "Algorithm"() -> (w333:T8)
                  n194 = local read "AlgParameter"() -> (w330:string)
                  n195 = control-ref of="List ROI"() -> (w329:refnum<vi>)
                  n196 = call "Imaq GetImageInfo"("Image"=w316) -> ("Image Type"=w332:T24)  [unwired: 3 in, 7 out]
                  n197 = Index Array(array=w322, index (row)=w321, index (col)=2 ("disabled index (col)")) -> (element=w319:string)
                  n198 = local read "Root Path"() -> (w327:path)
                  n199 = call "IMAQ Create"("Image Name"="SetAlgPanel", "Image Type"=w332) -> ("New Image"=w317:T7)  [unwired: 3 in, 1 out]
                  n200 = property on="Image" class="ImageControl"() -> ("ROI"=w318:T25)  [unwired: 2 in, 2 out]
                  n201 = call "From JSON Text.vim"("Data Type and Default Value"=w318, "JSON"=w319) -> ("Data out"=w315:T25)  [unwired: 8 in, 1 out]
                  n202 = call-poly "IMAQ Extract Tetragon"("ROI Descriptor"=w315, "Image Dst"=w317, "Image Src"=w316) -> ("Image Dst Out"=w314:T7)  [unwired: 7 in, 1 out]
                  n203 = case shown="\"B_Area Check\"" w333 {
                    selector: w333 -> [_ w341 w349 _ w361 w367]
                    tunnel: w314 -> [_ w343 w351 w355 w363 w369]
                    tunnel: w330 -> [_ w337 w345 w352 w357 w364]
                    tunnel: w329 -> [_ w342 w350 _ w362 w368]
                    tunnel: w328 -> [_ w340 w348 _ w360 _]
                    tunnel: w327 -> [_ w339 w344 _ w356 _]
                    tunnel: [w334 w337 w345 w352 w357 w364] -> w323
                    tunnel: [FALSE ("Cancel?") w338 w346 w354 w358 w365] -> w326
                    tunnel: [w334 w336 w347 w353 w359 w366] -> w324
                    frame "None", Default {
                      w334 = "" ("AlgParameter")
                    }
                    frame "C_Color Pattern Matching" {
                      n204 = call "ColorPatternMatch_Setting_UI.vi"("Vision_Image In"=w343, "List ROI 2"=w342, "AlgIn"=w341, "ProjectName"=w340, "Parameter"=w337, "RootPath"=w339) -> ("Analysis_Setting"=w336:string, "Cancel?"=w338:bool)  [unwired: 7 in, 1 out]
                    }
                    frame "G_PatternMatching" {
                      n205 = call "PatternMatch_Setting_UI.vi"("Vision_Image In"=w351, "List ROI Ref"=w350, "AlgIn"=w349, "ProjectName"=w348, "ParameterIn"=w345, "RootPath"=w344) -> ("ParameerOut"=w347:string, "Cancel?"=w346:bool)  [unwired: 7 in, 1 out]
                    }
                    frame "G_ShapeDectect" {
                      n206 = call "ShapeDetect_Setting_UI.vi"("ParameterIn"=w352, "Vision_Image"=w355) -> ("Cancel?"=w354:bool, "ParameterOut"=w353:string)  [unwired: 7 in, 1 out]
                    }
                    frame "G_GeometricMatch" {
                      n207 = call "GeometricPatternMatch_Setting_UI.vi"("Vision_Image In"=w363, "List ROI Ref"=w362, "AlgIn"=w361, "ProjectName"=w360, "ParameterIn"=w357, "RootPath"=w356) -> ("ParameerOut"=w359:string, "IMAQ Curve Parameters.ctlCancel?"=w358:bool)  [unwired: 7 in, 1 out]
                    }
                    frame "B_Area Check" {
                      n208 = call "AreaCheck.vi"("Vision_Image In"=w369, "List ROI Ref"=w368, "AlgIn"=w367, "ParameterIn"=w364) -> ("ParameerOut"=w366:string, "Cancel?"=w365:bool)  [unwired: 9 in, 1 out]
                    }
                  }
                  n209 = property on="Algorithm" class="Enum (strict)"() -> ("RingText.Text"=w313:string)  [unwired: 2 in, 2 out]
                  n210 = Select(t=w323, s=w326, f=w324) -> (s? t:f=w325:string)
                  n211 = local write "AlgParameter"(w325) -> ()
                }
                frame "ShowPanel" {
                  n212 = local read "Image 2"() -> (w386:T7)
                  n213 = property on="Process List" class="MCListbox (strict)"() -> ("ItemNames"=w382:string[][], "Value"=w381:i32)  [unwired: 2 in, 2 out]
                  n214 = Index Array(array=w382, index (row) #1=w381, index (col) #1=2 ("disabled index (col)"), index (row) #2=w381, index (col) #2=1 ("disabled index (col)")) -> (element #1=w373:string, element #2=w383:string)
                  n215 = Decimal String To Number(string=w383) -> (number=w378:i32)  [unwired: 2 in, 1 out]
                  n216 = flat-sequence {
                    tunnel: w378 -> [w387]
                    tunnel: [w388] -> w377
                    frame #0 {
                      "PreProcess2" <- w387
                    }
                    frame #1 {
                      n217 = local read "PreProcess2"() -> (w388:T5)
                    }
                  }
                  n218 = property on="相機" class="Ring (strict)"() -> ("RingText.Text"=w372:string)  [unwired: 2 in, 2 out]
                  n219 = case shown="Default" w377 {
                    selector: w377 -> [_ w395]
                    tunnel: w386 -> [_ w397]
                    tunnel: w373 -> [w390 w396]
                    tunnel: [w392 w393] -> w376
                    tunnel: [w391 w394] -> w375
                    tunnel: w372 -> [w389 _]
                    frame "CamAttributes" {
                      n220 = call "camera attribute.vi"("ParameterIn"=w390, "CamName"=w389) -> ("Btn_Cancel 2"=w392:bool, "DataOut"=w391:string)  [unwired: 8 in]
                    }
                    frame Default {
                      n221 = call "Process_Setting_UI2.vi"("Image In"=w397, "PreProcess"=w395, "DataIn"=w396) -> ("ExitFLG"=w393:bool, "DataOut"=w394:string)  [unwired: 7 in]
                    }
                  }
                  n222 = Select(t=w373, s=w376, f=w375) -> (s? t:f=w374:string)
                  n223 = Replace Array Subset(array=w382, new element=w374, index (row)=w381, index (col)=2 ("disabled index (col)")) -> (w379:string[][])
                  n224 = property on="Process List" class="MCListbox (strict)"("ItemNames"=w379) -> (error out=w370:errorcluster)  [unwired: 2 in, 1 out]
                  n225 = property on="PreProcess2" class="Enum (strict)"(error in=w370) -> ("RingText.Text"=w371:string)  [unwired: 1 in, 2 out]
                }
                frame "Snap" {
                  n226 = local read "相機"() -> (w411:u16)
                  n227 = call "[FGV] Camera Settings.vi"("Action"=T20."Grab", "Value"=w411) -> ("error out"=w409:errorcluster, "Image Out"=w404:T7)  [unwired: 7 in, 1 out]
                  n228 = call "[FGV]Parameters.vi"("Parameter"=Parameter."Read") -> ("ParameterData Out"=w406:T27)  [unwired: 9 in, 1 out]
                  n229 = Unbundle By Name(w406) -> ("Cal?"=w405:bool, "Calibration File Path"=w403:string)
                  n230 = case shown="True" w405 {
                    tunnel: w404 -> [w412 w414]
                    tunnel: w403 -> [_ w415]
                    tunnel: [w412 w413] -> w402
                    frame False {
                    }
                    frame True {
                      n231 = call "IMAQ Set Calibration Info"("Image Dst"=w414, "Image Src"=w415) -> ("Calibrated Image"=w413:T7)  [unwired: 8 in, 1 out]
                    }
                  }
                  n232 = property on="相機" class="Ring (strict)"() -> ("RingText.Text"=w398:string)  [unwired: 2 in, 2 out]
                  n233 = call "IMAQ Copy"("Image Dst"="oringal" ("Image Name"), "Image Src"=w402) -> ("Image Dst Out"=w399:T7)  [unwired: 4 in, 1 out]
                  n234 = call "IMAQ Get Calibration Info 3"("Calibration Template Image"=w399) -> ("Grid Descriptor"=→"Grid Descriptor":T3, "Calibration Axis Info"=→"Calibration Axis Info":T2)  [unwired: 6 in, 7 out]
                  n235 = local write "Image"(w402) -> ()
                }
                frame "UpDateDataToList ROI" {
                  n236 = local read "ProjectSet"() -> (w419:u16)
                  n237 = call "[FGV]VParameters.vi"("Enum"=T17."Read", "ProjectIndex"=w419) -> ("DataOut"=w418:T16)  [unwired: 6 in, 3 out]
                  n238 = Unbundle(w418) -> ("Parameter"=w417:string[][])  [unwired: 1 out]
                  n239 = property on="List ROI" class="MCListbox (strict)"("ItemNames"=w417) -> ()  [unwired: 2 in, 2 out]
                }
                frame "UpDateDataToProcess" {
                  n240 = property on="List ROI" class="MCListbox (strict)"() -> ("ItemNames"=w449:string[][], "Value"=w427:i32)  [unwired: 2 in, 2 out]
                  n241 = Index Array(array=w449, index (row) #1=w427, index (col) #1=3 ("disabled index (col)"), index (row) #2=w427, index (col) #2=4 ("disabled index (col)"), index (row) #3=w427, index (col) #3=5 ("disabled index (col)"), index (row) #4=w427, index (col) #4=6 ("disabled index (col)")) -> (element #1=w447:string, element #2=w440:string, element #3=w439:string, element #4=w423:string)
                  n242 = call "From JSON Text.vim"("Data Type and Default Value"=string[][] [], "JSON"=w447) -> ("error out"=w438:errorcluster, "Data out"=w445:string[][])  [unwired: 8 in]
                  n243 = call "From JSON Text.vim"("Data Type and Default Value"=string[] [], "JSON"=w440) -> ("error out"=w437:errorcluster, "Data out"=w433:string[])  [unwired: 8 in]
                  n244 = call "From JSON Text.vim"("Data Type and Default Value"=string[][] [], "JSON"=w439) -> ("error out"=w436:errorcluster, "Data out"=w428:string[][])  [unwired: 8 in]
                  n245 = call "From JSON Text.vim"("Data Type and Default Value"=string[][] [], "JSON"=w423) -> ("error out"=w422:errorcluster, "Data out"=w424:string[][])  [unwired: 8 in]
                  n246 = Index Array(array=w433, index #1=1 ("index")) -> (element #1=w430:string, element #2=w431:string)  [unwired: 1 in]
                  n247 = property on="Process List" class="MCListbox (strict)"("ItemNames"=w445) -> ()  [unwired: 2 in, 2 out]
                  n248 = property on="OutPutList" class="MCListbox (strict)"("ItemNames"=w424) -> ()  [unwired: 2 in, 2 out]
                  n249 = property on="Result" class="MCListbox (strict)"("ItemNames"=w428) -> ()  [unwired: 2 in, 2 out]
                  n250 = Decimal String To Number(string=w430) -> (number=w429:i32)  [unwired: 2 in, 1 out]
                  n251 = local write "AlgParameter"(w431) -> ()
                  n252 = local write "Algorithm"(w429) -> ()
                  n253 = Merge Errors(w438, w437, w436, w422) -> (w435:errorcluster)
                  n254 = call <vilib>:"Clear Errors.vi"("error in (no error)"=w435) -> ("error out"=w434:errorcluster)  [unwired: 5 in, 1 out]
                }
                frame "UpdateProjectSet" {
                  n255 = call "[FGV]VParameters.vi"("Enum"=T17."ReadProjectName") -> ("ProjectName"=w451:string[])  [unwired: 7 in, 3 out]
                  n256 = property on="ProjectSet" class="Ring (strict)"("Strings []"=w451) -> ()  [unwired: 2 in, 2 out]
                }
                frame "WriteToDataTable" {
                  n257 = property on="ProjectSet" class="Ring (strict)"() -> ("RingText.Text"=w453:string, "Value"=w452:u16)  [unwired: 2 in, 2 out]
                  n258 = property on="List ROI" class="MCListbox (strict)"() -> ("ItemNames"=w454:string[][])  [unwired: 2 in, 2 out]
                  n259 = Bundle("RingText.Text"=w453, "ItemNames"=w454) -> (w455:T28)  [unwired: 1 in]
                  n260 = call "[FGV]VParameters.vi"("Enum"=T17."write", "ProjectIndex"=w452, "DataIn"=w455) -> ()  [unwired: 5 in, 4 out]
                }
                frame "exit" {
                  n261 = call "IMAQ Dispose"("All Images? (No)"=TRUE) -> ()  [unwired: 5 in, 1 out]
                  n262 = call "[FGV] Camera Settings.vi"("Action"=T20."Close") -> ()  [unwired: 8 in, 3 out]
                  n263 = call "Exit.vi"("Enum"=enum16{"Initial", "Read", "Write"}."Read") -> ("ExitOut"=w459:bool)  [unwired: 10 in]
                }
              }
              n264 = case shown="Error .." w30 {
                selector: w30 -> [_ w46]
                tunnel: w27 -> [w37 _]
                tunnel: w26 -> [w34 _]
                frame No Error {
                  n265 = Concatenate Strings(w37, "," ("string"), w34) -> (w36:string)
                  n266 = Bundle By Name(cluster=T13 {"MsgPageSelect"=enum."Action", "LogType"=enum."Manual", "Msg"="", "Time"=""} ("DataIn"), "Msg"=w36) -> (w39:T13)
                  n267 = call "SendMsg.vi"("DataIn"=w39) -> ()  [unwired: 10 in, 1 out]
                }
                frame Error {
                  n268 = Unbundle By Name(w46) -> ("source"=w41:string, "code"=w40:i32)
                  n269 = Format Into String(format string="ErrorCode:%d_ErrorMsg:%s", w40, w41) -> (resulting string=w42:string)  [unwired: 2 in, 1 out]
                  n270 = One Button Dialog(message=w41) -> ()  [unwired: 1 in, 1 out]
                  n271 = Bundle By Name(cluster=T13 {"MsgPageSelect"=enum."Alarm", "LogType"=enum."Auto", "Msg"="", "Time"=""} ("DataIn"), "Msg"=w42) -> (w44:T13)
                  n272 = call "SendMsg.vi"("DataIn"=w44) -> ()  [unwired: 10 in, 1 out]
                }
              }
            }
          }
          frame True {
            n273 = case shown="True" "btn_Grab" {
              frame False {
              }
              frame True {
                n274 = local read "相機"() -> (w476:u16)
                n275 = call "[FGV]Parameters.vi"("Parameter"=Parameter."Read") -> ("ParameterData Out"=w475:T27)  [unwired: 9 in, 1 out]
                n276 = call "[FGV] Camera Settings.vi"("Action"=T20."Grab", "Value"=w476) -> ("Image Out"=w473:T7)  [unwired: 7 in, 2 out]
                n277 = Unbundle By Name(w475) -> ("Cal?"=w474:bool, "Calibration File Path"=w472:string)
                n278 = case shown="True" w474 {
                  tunnel: w473 -> [w477 w479]
                  tunnel: w472 -> [_ w480]
                  tunnel: [w477 w478] -> w471
                  frame False {
                  }
                  frame True {
                    n279 = call "IMAQ Set Calibration Info"("Image Dst"=w479, "Image Src"=w480) -> ("Calibrated Image"=w478:T7)  [unwired: 8 in, 1 out]
                  }
                }
                n280 = call "IMAQ Copy"("Image Dst"="oringal" ("Image Name"), "Image Src"=w471) -> ()  [unwired: 4 in, 2 out]
                n281 = local write "Image"(w471) -> ()
              }
            }
            n282 = property on="List ROI" class="MCListbox (strict)"() -> ("Value"=w465:i32)  [unwired: 2 in, 2 out]
            n283 = Less Than 0?(x=w465) -> (x < 0?=w464:bool)
            n284 = Select(t=T22."Disabled and Grayed Out" ("Disabled"), s=w464, f=T22."Enabled") -> (s? t:f=w461:T22)
            n285 = property on="Btn_RenewROIData" class="Bool"("DisabledEnum"=w461) -> ()  [unwired: 2 in, 2 out]
            n286 = property on="Tab Control 2" class="TabCtl (strict)"("DisabledEnum"=w461) -> ()  [unwired: 2 in, 2 out]
          }
        }
      }
      n287 = while {
        tunnel: w16 -> [w482]
        tunnel: [w481] -> w15
        stop <- w484 stop-if-true
        n288 = event shown="[17] \"Btn_Test\": Value Change" {
          selector: _ -> [_ _ _ _ _ _ _ _ _ _ _ _ _ _ _ _ _ _ _ _ _ _ _ _]
          dyn-events: _ -> [_ _ _ _ _ _ _ _ _ _ _ _ _ _ _ _ _ _ _ _ _ _ _ _]
          timeout: 500 -> [_ _ _ _ _ _ _ _ _ _ _ _ _ _ _ _ _ _ _ _ _ _ _ _]
          tunnel: [_ _ _ _ _ _ _ _ _ _ _ _ _ _ _ _ _ _ _ _ _ _ _ w591] -> w484
          tunnel: w482 -> [_ w490 w492 w494 _ w503 _ _ w522 w524 w526 w528 w529 w540 w542 w550 w552 w556 w567 w569 w571 w573 w588 w589]
          tunnel: [_ _ _ _ _ _ _ _ _ _ _ _ _ _ _ _ _ _ _ _ _ _ _ w589] -> w481
          event Value Change {
            n289 = event-data() -> ("NewVal"=w487:T8)  [unwired: 1 in, 5 out]
            n290 = Equal?(x=w487, y=V_Analysis_Type."None") -> (x = y?=w485:bool)
            n291 = case shown="False" w485 {
              frame False {
              }
              frame True {
                n292 = local write "AlgParameter"("") -> ()
              }
            }
          }
          event "Btn_Add PreProcess": Value Change {
            n293 = event-data() -> ()  [unwired: 1 in, 1 out]
            n294 = Lossy Enqueue Element(queue=w490, element=cluster{"Action":string, "Varient":variant}[] [{"Action"="Add PreProcess", "Varient"=variant}]) -> ()  [unwired: 1 in, 4 out]
          }
          event "Btn_AddProject": Value Change {
            n295 = event-data() -> ()  [unwired: 1 in, 1 out]
            n296 = Lossy Enqueue Element(queue=w492, element=cluster{"Action":string, "Varient":variant}[] [{"Action"="AddProject", "Varient"=variant}, {"Action"="UpdateProjectSet", "Varient"=variant}]) -> ()  [unwired: 1 in, 4 out]
          }
          event "Btn_AddROI": Value Change {
            n297 = event-data() -> ()  [unwired: 1 in, 1 out]
            n298 = Lossy Enqueue Element(queue=w494, element=cluster{"Action":string, "Varient":variant}[] [{"Action"=" AddROI", "Varient"=variant}]) -> ()  [unwired: 1 in, 4 out]
          }
          event Value Change {
            n299 = event-data() -> ()  [unwired: 1 in, 6 out]
            n300 = local read "Root Path"() -> (w501:path)
            n301 = call "Calibration_Setting_UI.vi"("Real Position Info"=T23 {"Real Points Valid?"=FALSE, "Real Position"=[]}, "CamGot?"=TRUE, "Cal Info Image"=T7 refnum, "Cal Status In"=FALSE, "Root Path"=w501, "Seq"="") -> ("Calibration Done"=→"Calibration Done":bool)  [unwired: 3 in, 2 out]
          }
          event "Btn_DelProject": Value Change {
            n302 = event-data() -> ()  [unwired: 1 in, 3 out]
            n303 = Enqueue Element(queue=w503, element=cluster{"Action":string, "Varient":variant}[] [{"Action"="DelProject", "Varient"=variant}]) -> ()  [unwired: 2 in, 3 out]
          }
          event "Btn_DelROI": Value Change {
            n304 = event-data() -> ()  [unwired: 1 in, 2 out]
            n305 = property on="List ROI" class="MCListbox (strict)"() -> ("ItemNames"=w509:string[][], "Value"=w508:i32)  [unwired: 2 in, 2 out]
            n306 = Index Array(array=w509, index (row)=w508, index (col)=0 ("disabled index (col)")) -> (element=w506:string)
            n307 = Format Into String(format string="確認是否刪除%s設定\nMake Sure Delete %s", w506, w506) -> (resulting string=w505:string)  [unwired: 2 in, 1 out]
            n308 = Two Button Dialog(message=w505) -> (T button?=w504:bool)  [unwired: 2 in]
            n309 = case shown="True" w504 {
              tunnel: w509 -> [_ w514]
              tunnel: w508 -> [_ w513]
              frame False {
              }
              frame True {
                n310 = Delete From Array(array=w514, length=1, index (row)=w513) -> (array with subset deleted=w512:string[][])  [unwired: 1 in, 1 out]
                n311 = property on="List ROI" class="MCListbox (strict)"("ItemNames"=w512) -> ()  [unwired: 2 in, 2 out]
              }
            }
          }
          event "Btn_EditROI": Value Change {
            (unwired) T29 {"Global Rectangle"=[], "Contours"=[]}  # ROI Descriptor
            n312 = event-data() -> ()  [unwired: 1 in, 3 out]
            n313 = property on="Image" class="ImageControl"() -> ("ROI"=w516:T25)  [unwired: 2 in, 2 out]
            n314 = property on="List ROI" class="MCListbox (strict)"() -> ("ItemNames"=w520:string[][], "Value"=w518:i32)  [unwired: 2 in, 2 out]
            n315 = call "To JSON Text.vim"("Anything"=w516) -> ("<JSON>"=w515:string)  [unwired: 9 in, 1 out]
            n316 = Replace Array Subset(array=w520, new element=w515, index (row)=w518, index (col)=2 ("disabled index (col)")) -> (w519:string[][])
            n317 = property on="List ROI" class="MCListbox (strict)"("ItemNames"=w519) -> ()  [unwired: 2 in, 2 out]
          }
          event "Btn_Load": Value Change {
            n318 = event-data() -> ()  [unwired: 1 in, 1 out]
            n319 = Enqueue Element(queue=w522, element=cluster{"Action":string, "Varient":variant}[] [{"Action"="UpDateDataToUI", "Varient"=variant}]) -> ()  [unwired: 2 in, 3 out]
          }
          event "Btn_RemovePreProcess": Value Change {
            n320 = event-data() -> ()  [unwired: 1 in, 1 out]
            n321 = Lossy Enqueue Element(queue=w524, element=cluster{"Action":string, "Varient":variant}[] [{"Action"="RemovePreProcess", "Varient"=variant}]) -> ()  [unwired: 1 in, 4 out]
          }
          event Value Change {
            n322 = event-data() -> ()  [unwired: 1 in, 1 out]
            n323 = Enqueue Element(queue=w526, element=cluster{"Action":string, "Varient":variant}[] [{"Action"="RenewROIData", "Varient"=variant}, {"Action"="Clear ChangeProject", "Varient"=variant}]) -> ()  [unwired: 2 in, 3 out]
          }
          event "Btn_ResultAdd": Value Change {
            n324 = event-data() -> ()  [unwired: 1 in, 1 out]
            n325 = Enqueue Element(queue=w528, element=cluster{"Action":string, "Varient":variant}[] [{"Action"="ResultAdd", "Varient"=variant}]) -> ()  [unwired: 2 in, 3 out]
          }
          event "Btn_Result Remove": Value Change {
            n326 = event-data() -> ()  [unwired: 1 in, 1 out]
            n327 = property on="OutPutList" class="MCListbox (strict)"() -> ("ItemNames"=w536:string[][], "Value"=w535:i32)  [unwired: 2 in, 2 out]
            n328 = Index Array(array=w536, index (row)=w535, index (col)=0 ("disabled index (col)")) -> (element=w532:string)
            n329 = Format Into String(format string="確認是否刪除輸出資料%s?\nMake Sure Delete Output Parameter %s?", w532, w532) -> (resulting string=w531:string)  [unwired: 2 in, 1 out]
            n330 = Two Button Dialog(message=w531) -> (T button?=w530:bool)  [unwired: 2 in]
            n331 = case shown="True" w530 {
              tunnel: w529 -> [_ w538]
              frame False {
              }
              frame True {
                n332 = Enqueue Element(queue=w538, element=cluster{"Action":string, "Varient":variant}[] [{"Action"="DeleteOutPutList", "Varient"=variant}]) -> ()  [unwired: 2 in, 3 out]
              }
            }
          }
          event "Btn_ROITryrun": Value Change {
            n333 = event-data() -> ()  [unwired: 1 in, 1 out]
            n334 = Enqueue Element(queue=w540, element=cluster{"Action":string, "Varient":variant}[] [{"Action"="RunROIList", "Varient"=variant}]) -> ()  [unwired: 2 in, 3 out]
          }
          event "Btn_Save": Value Change {
            n335 = event-data() -> ()  [unwired: 1 in, 2 out]
            n336 = Lossy Enqueue Element(queue=w542, element=cluster{"Action":string, "Varient":variant}[] [{"Action"="WriteToDataTable", "Varient"=variant}, {"Action"="SaveDataTable", "Varient"=variant}]) -> ()  [unwired: 1 in, 4 out]
          }
          event "Btn_SetAlg": Value Change {
            n337 = event-data() -> ()  [unwired: 1 in, 2 out]
            n338 = property on="Process List" class="MCListbox (strict)"() -> ("ItemNames"=w545:string[][])  [unwired: 2 in, 2 out]
            n339 = Array Size(array=w545) -> (size(s)=w544:i32[])
            n340 = Index Array(array=w544) -> (element=w543:i32)  [unwired: 1 in]
            n341 = Bundle By Name(cluster=cluster{"Action":string, "Varient":variant} {"Action"=" RunProcess", "Varient"=variant}, "Varient"=w543) -> (w546:cluster{"Action":string, "Varient":variant})
            n342 = Build Array(w546, cluster{"Action":string, "Varient":variant} {"Action"="SetAlgPanel", "Varient"=variant}) -> (w547:cluster{"Action":string, "Varient":variant}[])
            n343 = Enqueue Element(queue=w550, element=w547) -> ()  [unwired: 2 in, 3 out]
          }
          event Value Change {
            n344 = event-data() -> ()  [unwired: 1 in, 3 out]
            n345 = Lossy Enqueue Element(queue=w552, element=cluster{"Action":string, "Varient":variant}[] [{"Action"="Snap", "Varient"=variant}]) -> ()  [unwired: 1 in, 4 out]
          }
          event "Btn_Test": Value Change {
            n346 = event-data() -> ()  [unwired: 1 in, 2 out]
            n347 = property on="Process List" class="MCListbox (strict)"() -> ("ItemNames"=w555:string[][])  [unwired: 2 in, 2 out]
            n348 = Array Size(array=w555) -> (size(s)=w554:i32[])
            n349 = Index Array(array=w554) -> (element=w553:i32)  [unwired: 1 in]
            n350 = Bundle By Name(cluster=cluster{"Action":string, "Varient":variant} {"Action"=" RunProcess", "Varient"=variant}, "Varient"=w553) -> (w559:cluster{"Action":string, "Varient":variant})
            n351 = Build Array(w559) -> (w558:cluster{"Action":string, "Varient":variant}[])
            n352 = Enqueue Element(queue=w556, element=w558) -> ()  [unwired: 2 in, 3 out]
          }
          event "Btn_TestAlg": Value Change {
            n353 = event-data() -> ()  [unwired: 1 in, 2 out]
            n354 = property on="Process List" class="MCListbox (strict)"() -> ("ItemNames"=w562:string[][])  [unwired: 2 in, 2 out]
            n355 = Array Size(array=w562) -> (size(s)=w561:i32[])
            n356 = Index Array(array=w561) -> (element=w560:i32)  [unwired: 1 in]
            n357 = Bundle By Name(cluster=cluster{"Action":string, "Varient":variant} {"Action"=" RunProcess", "Varient"=variant}, "Varient"=w560) -> (w563:cluster{"Action":string, "Varient":variant})
            n358 = Build Array(w563, cluster{"Action":string, "Varient":variant} {"Action"="RunAlg", "Varient"=variant}) -> (w564:cluster{"Action":string, "Varient":variant}[])
            n359 = Enqueue Element(queue=w567, element=w564) -> ()  [unwired: 2 in, 3 out]
          }
          event "List ROI": Mouse Down {
            n360 = event-data() -> ()  [unwired: 1 in, 1 out]
            n361 = Enqueue Element(queue=w569, element=cluster{"Action":string, "Varient":variant}[] [{"Action"="UpDateDataToProcess", "Varient"=variant}, {"Action"="OverlayROI", "Varient"=variant}]) -> ()  [unwired: 2 in, 3 out]
          }
          event Value Change {
            n362 = event-data() -> ()  [unwired: 1 in, 1 out]
            n363 = Enqueue Element(queue=w571, element=cluster{"Action":string, "Varient":variant}[] [{"Action"="Photo", "Varient"=variant}]) -> ()  [unwired: 2 in, 3 out]
          }
          event "Process List": Mouse Down {
            n364 = event-data() -> ("Mods.Double Click"=w574:bool)  [unwired: 1 in, 3 out]
            n365 = property on="Process List" class="MCListbox (strict)"() -> ("Value"=w572:i32)  [unwired: 2 in, 2 out]
            n366 = case shown="False" w574 {
              tunnel: w573 -> [w579 w586]
              tunnel: w572 -> [w575 w580]
              frame False {
                n367 = Bundle By Name(cluster=cluster{"Action":string, "Varient":variant} {"Action"=" RunProcess", "Varient"=variant}, "Varient"=w575) -> (w577:cluster{"Action":string, "Varient":variant})
                n368 = Build Array(w577) -> (w576:cluster{"Action":string, "Varient":variant}[])
                n369 = Enqueue Element(queue=w579, element=w576) -> ()  [unwired: 2 in, 3 out]
              }
              frame True {
                n370 = Bundle By Name(cluster=cluster{"Action":string, "Varient":variant} {"Action"=" RunProcess", "Varient"=variant}, "Varient"=w580) -> (w583:cluster{"Action":string, "Varient":variant})
                n371 = Bundle By Name(cluster=cluster{"Action":string, "Varient":variant} {"Action"="ShowPanel", "Varient"=variant}, "Varient"=w580) -> (w582:cluster{"Action":string, "Varient":variant})
                n372 = Build Array(w583, w582) -> (w581:cluster{"Action":string, "Varient":variant}[])
                n373 = Enqueue Element(queue=w586, element=w581) -> ()  [unwired: 2 in, 3 out]
              }
            }
          }
          event "ProjectSet": Value Change {
            # "CamAttributes"
            n374 = event-data() -> ()  [unwired: 1 in, 6 out]
            n375 = Lossy Enqueue Element(queue=w588, element=cluster{"Action":string, "Varient":variant}[] [{"Action"="UpDateDataToList ROI", "Varient"=variant}, {"Action"="Clear ChangeProject ", "Varient"=variant}]) -> ()  [unwired: 1 in, 4 out]
          }
          event Timeout {
            n376 = event-data() -> ()  [unwired: 1 in, 3 out]
            n377 = call "Exit.vi"("Enum"=enum16{"Initial", "Read", "Write"}."Read") -> ("ExitOut"=w591:bool)  [unwired: 10 in]
          }
        }
      }
      n378 = Enqueue Element(queue=w15, element=cluster{"Action":string, "Varient":variant}[] [{"Action"="exit", "Varient"=variant}]) -> ()  [unwired: 2 in, 3 out]
    }
  }
